vi "Get Image Data.vi"(0 "fpga interface in":refnum<k20>, 1 "'stop' notifier":refnum<notifier>, 5 "display channel number":i32, 7 "raw display notifier":refnum<notifier>, 11 "error in (no error)":errorcluster) -> (4 "fpga interface out":refnum<k20>, 6 "output cluster":T3, 8 "output cluster 2":T2, 15 "error out":errorcluster)   [LabVIEW 2026]
uses:
  Types/Serial Channel Display Parameters.ctl
  <vilib>/vision/Image Controls.llb/IMAQ Image.ctl
  Types/RAW Interpretation for Display.ctl
  Types/148x_Common_FPGA_Reference.ctl
  <vilib>/Utility/error.llb/Error Cluster From Error Code.vi
  <vilib>/rvi/errors/niLvFpgaAdjustHostInterfaceError.vi
  <vilib>/rvi/interface/nirviReadWriteControl/nirviReadWriteControl.xnode
  GettingStarted_Common_148X_Host.lvlib
  NiFpgaLv.dll
  <vilib>/rvi/interface/Simulation/niFpgaSimulationCallBeginRW.vi
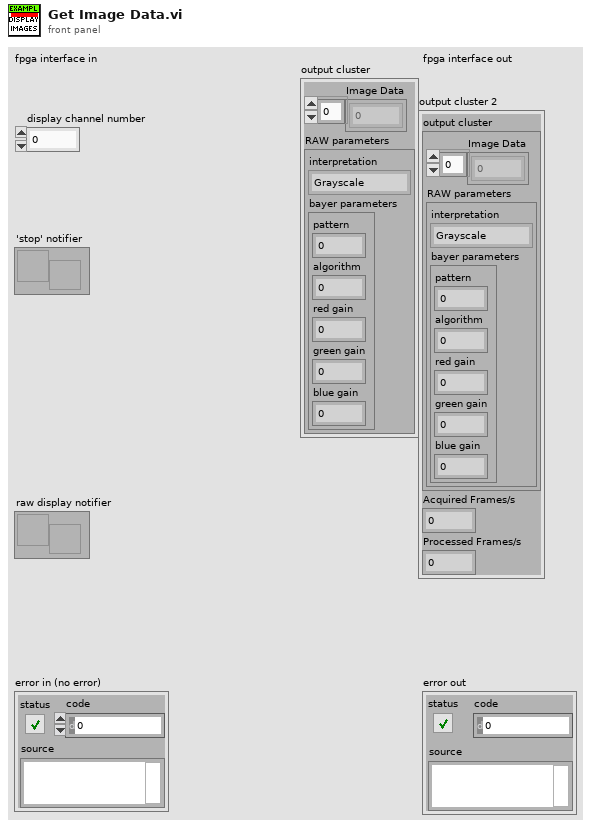
[diagram p1: front panel]
types:
  T1 = typedef "GettingStarted_Common_148X_Host.lvlib/RAW Interpretation for Display.ctl" = enum16{"Grayscale", "Bayer", "RGB", "YUV422", "YUV420", "Legacy YUV420"}
  T2 = cluster{"output cluster":cluster{"Image Data":u8[], "RAW parameters":cluster{"interpretation":T1, "bayer parameters":cluster{"pattern":i32, "algorithm":i32, "red gain":dbl, "green gain":dbl, "blue gain":dbl}}}, "Acquired Frames/s":dbl, "Processed Frames/s":dbl}
  T3 = cluster{"Image Data":u8[], "RAW parameters":cluster{"interpretation":T1, "bayer parameters":cluster{"pattern":i32, "algorithm":i32, "red gain":dbl, "green gain":dbl, "blue gain":dbl}}}
  T4 = typedef "GettingStarted_Common_148X_Host.lvlib/148x_Common_FPGA_Reference.ctl" = refnum<k20>
  T5 = typedef "GettingStarted_Common_148X_Host.lvlib/Serial Channel Display Parameters.ctl" = cluster{"images":cluster{"grayscale":T6, "color":T6}, "RAW parameters":cluster{"interpretation":T1, "bayer parameters":cluster{"pattern":i32, "algorithm":i32, "red gain":dbl, "green gain":dbl, "blue gain":dbl}}}
  T6 = typedef "IMAQ Image.ctl" = refnum<image>
  T7 = typedef "GettingStarted_Common_148X_FPGA.lvlib/Image Metadata.ctl" = cluster{"serial channel":fxp<+,3,3>, "frame number":u16, "data type":T8, "width":u16, "height":u16, "image bytes":u32, "total bytes":u32, "little endian":bool}
  T8 = typedef "NI CSI-2 API Common v2.lvlib/LLP Data Type.ctl" = enum8{"Frame Start", "Frame End", "Line Start", "Line End", "End of Transmission", "Reserved 0", "Reserved 1", "Reserved 2", "Generic Short Packet 1", "Generic Short Packet 2", "Generic Short Packet 3", "Generic Short Packet 4", "Generic Short Packet 5", "Generic Short Packet 6", "Generic Short Packet 7", "Generic Short Packet 8", "Null", "Blanking Data", "Embedded 8-bit non Image Data", "Generic Long Packet 1", "Generic Long Packet 2", "Generic Long Packet 3", "Generic Long Packet 4", "Reserved 3", "YUV420 8-bit", "YUV420 10-bit", "Legacy YUV420 8-bit", "Reserved 4", "YUV420 8-bit Chroma Shifted", "YUV420 10-bit Chroma Shifted", "YUV422 8-bit", "YUV422 10-bit", "RGB444", "RGB555", "RGB565", "RGB666", "RGB888", "Reserved 5", "Reserved 6", "RAW 24", "RAW 6", "RAW 7", "RAW 8", "RAW 10", "RAW 12", "RAW 14", "RAW 16", "RAW 20", "User Defined 8-bit Data 1", "User Defined 8-bit Data 2", "User Defined 8-bit Data 3", "User Defined 8-bit Data 4", "User Defined 8-bit Data 5", "User Defined 8-bit Data 6", "User Defined 8-bit Data 7", "User Defined 8-bit Data 8", "USL Command", "Reserved 7", "Reserved 8", "Reserved 9", "Reserved 10", "Reserved 11", "Reserved 12", "LRTE EPD Spacer"}
  T9 = cluster{"image pixel data fifo overflow":bool, "image metadata fifo overflow":bool}[]
  T10 = cluster{"image pixel data fifo overflow":bool, "image metadata fifo overflow":bool}
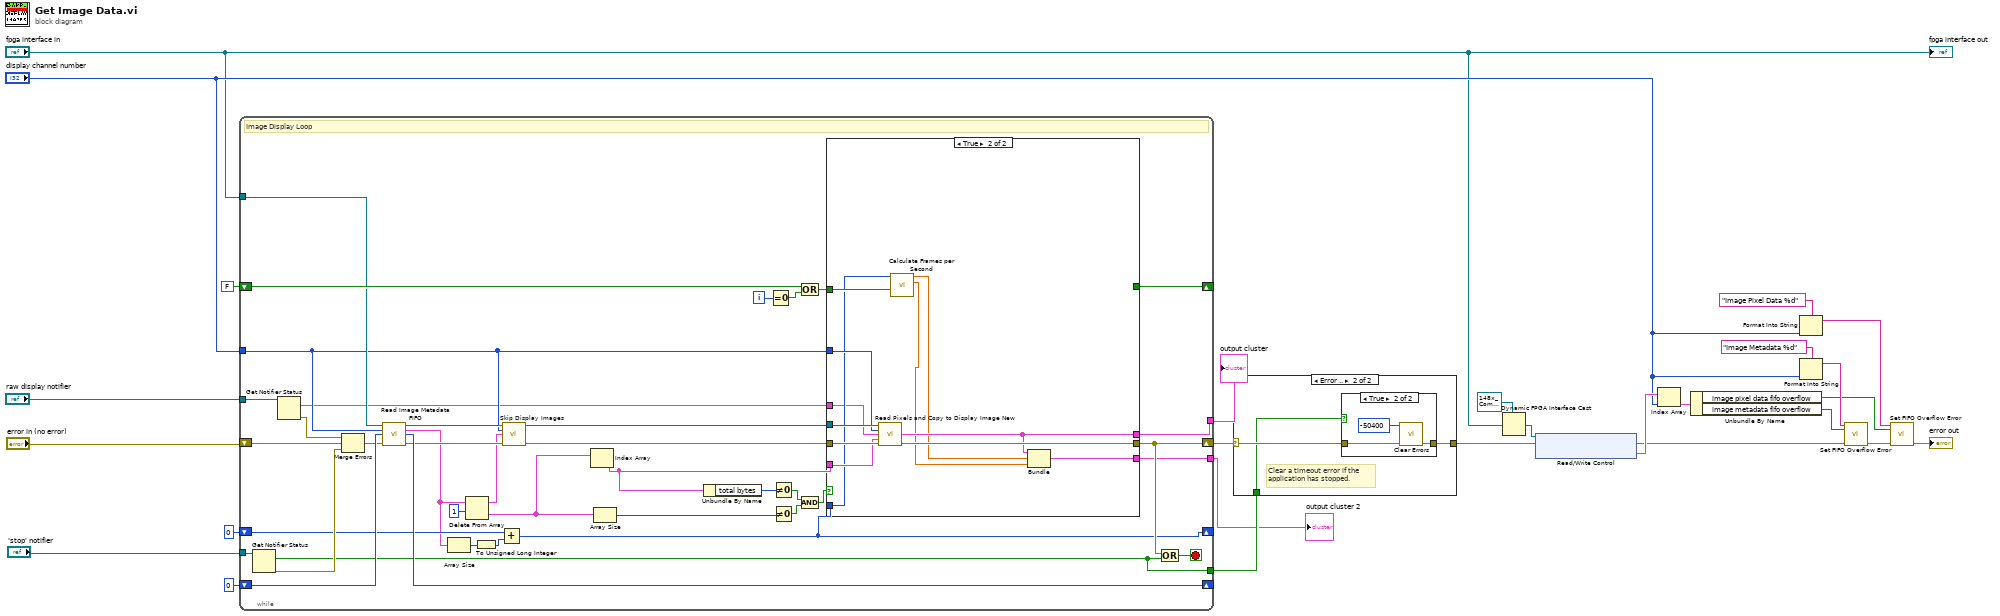
[diagram p0: block diagram]
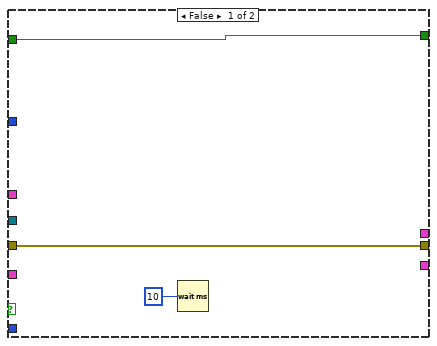
[diagram p2: hidden frame]
diagram:
  n1 = while {
    shift-right: [w62] -> w8
    shift-left: "error in (no error)" -> [w33]
    tunnel: "fpga interface in" -> [w37]
    shift-right: [w63] -> _
    shift-left: u32 0 ("Elements Remaining") -> [w51]
    tunnel: "display channel number" -> [w32]
    shift-right: [w55] -> _
    shift-left: FALSE -> [w52]
    shift-right: [w39] -> _
    shift-left: u32 0 ("Elements Remaining") -> [w42]
    tunnel: [w35] -> w5
    tunnel: "'stop' notifier" -> [w36]
    tunnel: "raw display notifier" -> [w31]
    tunnel: [w28] -> w2
    tunnel: [w27] -> w1
    i -> [w61]
    stop <- w64 stop-if-true
    # "Image Display Loop"
    n2 = Get Notifier Status(notifier=w36) -> (current notification=w35:bool, error out=w65:errorcluster)  [unwired: 1 in, 3 out]
    n3 = Get Notifier Status(notifier=w31) -> (current notification=w30:T5[], error out=w29:errorcluster)  [unwired: 1 in, 3 out]
    n4 = Merge Errors(w29, w33, w65) -> (w34:errorcluster)
    n5 = call "Read Image Metadata FIFO.vi"("fpga inteface in"=w37, "display channel number"=w32, "number of images"=w51, "error in (no error)"=w34) -> ("fpga interface out"=w47:refnum<k20>, "image metadata"=w38:T7[], "images remaining"=w63:u32, "error out"=w44:errorcluster)  [unwired: 8 in]
    n6 = Array Size(array=w38) -> (size(s)=w41:i32)
    n7 = Delete From Array(array=w38, length=1) -> (deleted portion=w48:T7[], array with subset deleted=w43:T7[])  [unwired: 1 in]
    n8 = To Unsigned Long Integer(number=w41) -> (unsigned 32bit integer=w40:u32)
    n9 = Add(x=w42, y=w40) -> (x+y=w39:u32)
    n10 = call "Skip Display Images.vi"("fpga interface in"=w47, "display channel number"=w32, "image metadata"=w43, "error in (no error)"=w44) -> ("fpga interface out"=w46:refnum<k20>, "error out"=w45:errorcluster)  [unwired: 10 in]
    n11 = Index Array(array=w48) -> (element=w60:T7)  [unwired: 1 in]
    n12 = Array Size(array=w48) -> (size(s)=w50:i32)
    n13 = Unbundle By Name(w60) -> ("total bytes"=w59:u32)
    n14 = Equal To 0?(x=w61) -> (x = 0?=w53:bool)
    n15 = Not Equal To 0?(x=w59) -> (x != 0?=w57:bool)
    n16 = Not Equal To 0?(x=w50) -> (x != 0?=w58:bool)
    n17 = Compound Arithmetic op=OR(w52, w53) -> (w54:bool)
    n18 = Compound Arithmetic op=AND(w57, w58) -> (w56:bool)
    n19 = case shown="True" w56 {
      tunnel: w45 -> [w68 w80]
      tunnel: w46 -> [_ w79]
      tunnel: w30 -> [_ w73]
      tunnel: w32 -> [_ w78]
      tunnel: [w68 w74] -> w62
      tunnel: w60 -> [_ w77]
      tunnel: w54 -> [w66 w76]
      tunnel: [w66 _] -> w55
      tunnel: w39 -> [_ w75]
      tunnel: [_ w72] -> w28
      tunnel: [_ w69] -> w27
      frame False {
        n20 = Wait (ms)(milliseconds to wait=u32 10) -> ()  [unwired: 1 out]
      }
      frame True {
        n21 = call "Read Pixels and Copy to Display Image New.vi"("fpga interface in"=w79, "display channel number"=w78, "serial channel display parameters"=w73, "image metadata"=w77, "error in (no error)"=w80) -> ("output cluster"=w72:T3, "error out"=w74:errorcluster)  [unwired: 7 in, 2 out]
        n22 = call <vilib>:"Calculate Frames per Second.vi"("Reset"=w76, "Buffer Number"=w75) -> ("Processed Frames/s"=w70:dbl, "Acquired Frames/s"=w71:dbl)  [unwired: 7 in, 1 out]
        n23 = Bundle("output cluster"=w72, "Acquired Frames/s"=w71, "Processed Frames/s"=w70) -> (w69:T2)  [unwired: 1 in]
      }
    }
    n24 = Compound Arithmetic op=OR(w62, w35) -> (w64:bool)
  }
  "output cluster" <- w2
  "output cluster 2" <- w1
  n25 = case shown="Error .." w8 {
    selector: w8 -> [w81 w84]
    tunnel: [w81 w83] -> w21
    tunnel: w5 -> [_ w82]
    frame No Error {
    }
    frame Error {
      # "Clear a timeout error if the application has stopped."
      n26 = case shown="True" w82 {
        tunnel: w84 -> [w85 w88]
        tunnel: [w85 w86] -> w83
        frame False {
        }
        frame True {
          n27 = call <vilib>:"Clear Errors.vi"("error in (no error)"=w88, "specific error code to clear (0: all)"=-50400 ("y")) -> ("error out"=w86:errorcluster)  [unwired: 4 in, 1 out]
        }
      }
    }
  }
  n28 = Dynamic FPGA Interface Cast(Session In=T4 refnum ("FPGA VI Reference Out"), Type="fpga interface in") -> (Session Out=w22:T4)
  n29 = xnode "Read/Write Control"("FPGA VI Reference In"=w22, "error in"=w21) -> ("error out"=w20:errorcluster, "display channel status"=w24:T9)  [unwired: 1 out]
  n30 = Index Array(array=w24, index="display channel number") -> (element=w25:T10)
  n31 = Unbundle By Name(w25) -> ("image pixel data fifo overflow"=w12:bool, "image metadata fifo overflow"=w11:bool)
  n32 = Format Into String(format string="Image Pixel Data %d", "display channel number") -> (resulting string=w14:string)  [unwired: 2 in, 1 out]
  n33 = Format Into String(format string="Image Metadata %d", "display channel number") -> (resulting string=w13:string)  [unwired: 2 in, 1 out]
  n34 = call "Set FIFO Overflow Error.vi"("fifo name"=w13, "overflow"=w11, "error in (no error)"=w20) -> ("error out"=w16:errorcluster)  [unwired: 12 in]
  n35 = call "Set FIFO Overflow Error.vi"("fifo name"=w14, "overflow"=w12, "error in (no error)"=w16) -> ("error out"=→"error out":errorcluster)  [unwired: 12 in]
  "fpga interface out" <- "fpga interface in"
